vi "CreateStageInfoFile.vi"(8 "error in (no error)":errorcluster, 9 "String":string, 10 "created path":path, 11 "GRMActor in":refnum<class "DataLoggerUI.lvclass">) -> (0 "error out":errorcluster, 1 "String dup":string, 2 "created path dup":path, 3 "GRMActor out":refnum<class "DataLoggerUI.lvclass">)   [LabVIEW 2020, in "DataLoggerUI.lvlib" / "DataLoggerUI.lvclass"]
uses:
  DataLoggerUI/DataLoggerUI.lvclass
  DataLoggerUI/DataLoggerUI.lvclass/DataLoggerUI.ctl
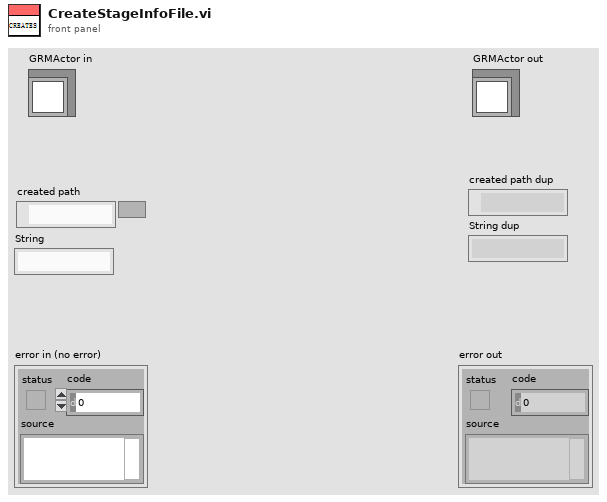
[diagram p1: front panel]
types:
  T1 = enum16{"open", "replace", "create", "open or create", "replace or create", "replace or create with confirmation"}
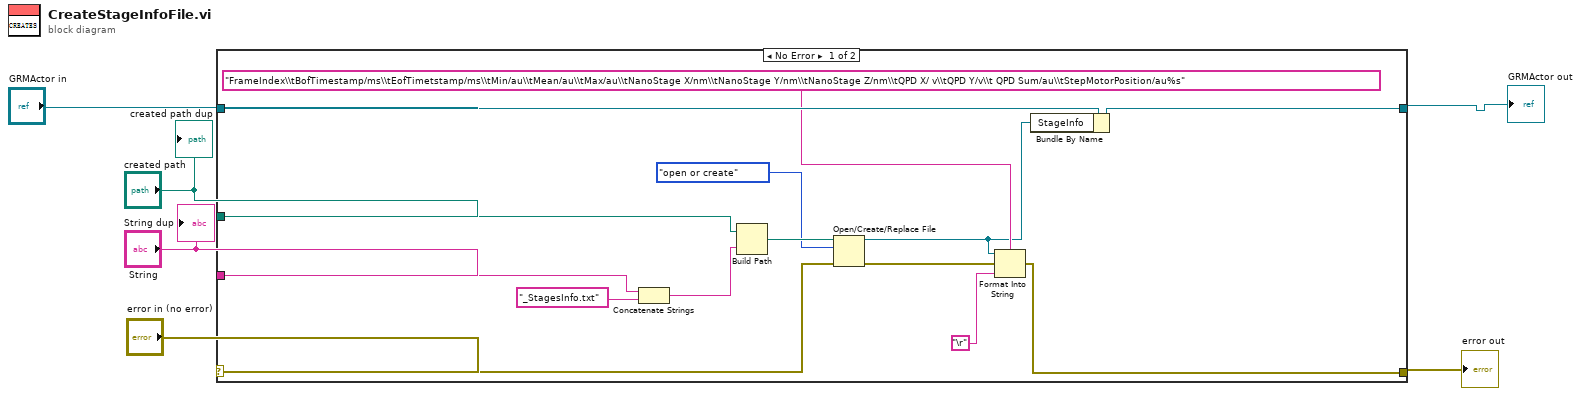
[diagram p0: block diagram]
diagram:
  n1 = case shown="No Error" "error in (no error)" {
    selector: "error in (no error)" -> [w15 w22]
    tunnel: [w9 w22] -> w3
    tunnel: [w12 w21] -> w1
    tunnel: "GRMActor in" -> [w13 w21]
    tunnel: "created path" -> [w17 _]
    tunnel: "String" -> [w19 _]
    frame No Error {
      n2 = Concatenate Strings(w19, "_StagesInfo.txt" ("string")) -> (w18:string)
      n3 = Build Path(base path=w17, name or relative path=w18) -> (appended path=w16:path)
      n4 = Open/Create/Replace File(file path (use dialog)=w16, error in=w15, operation (0:open)=T1."open or create") -> (refnum out=w7:refnum<file>, error out=w10:errorcluster)  [unwired: 3 in, 1 out]
      n5 = Format Into String(format string="FrameIndex\\tBofTimestamp/ms\\tEofTimetstamp/ms\\tMin/au\\tMean/au\\tMax/au\\tNanoStage X/nm\\tNanoStage Y/nm\\tNanoStage Z/nm\\tQPD X/ v\\tQPD Y/v\\t QPD Sum/au\\tStepMotorPosition/au%s" ("input 1"), initial string=w7, error in=w10, "\r") -> (error out=w9:errorcluster)  [unwired: 1 out]
      n6 = Bundle By Name(cluster=w13, "StageInfo"=w7) -> (w12:refnum<class "DataLoggerUI.lvclass">)
    }
    frame Error {
    }
  }
  "error out" <- w3
  "GRMActor out" <- w1
  "created path dup" <- "created path"
  "String dup" <- "String"
